vi "Read Port In.vi"(8 "error in (no error)":errorcluster caption="错误输入（无错误）", 10 "in_port":u16, 11 "dev":i32) -> (0 "error out":errorcluster caption="错误输出", 2 "in_port out":u16, 3 "function return":i32)   [LabVIEW 2018, in "恒凯采集卡.lvlib"]
doc: "int Read_Port_In(int dev,unsigned short* in_port);"
uses:
  data/Usb_Daq_V52_32.dll
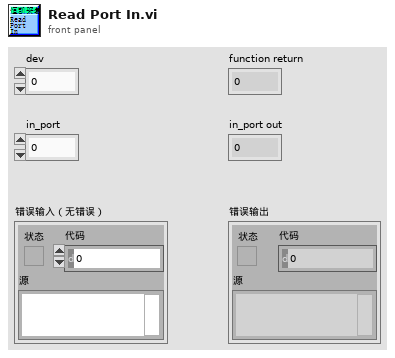
[diagram p1: front panel]
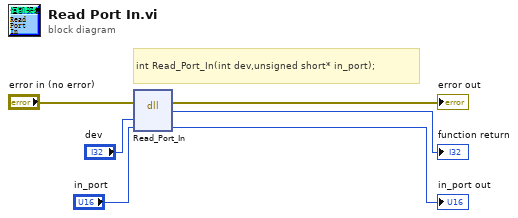
[diagram p0: block diagram]
diagram:
  # "int Read_Port_In(int dev,unsigned short* in_port);"
  n1 = dll-call lib="D:/ProgramFiles/NI/LabVIEW 2018/user.lib/Usb_Daq_V52_32/Usb_Daq_V52_32.*" fn="Read_Port_In"(error in="error in (no error)", "dev"="dev", "in_port"="in_port") -> (error out=→"error out":errorcluster, →"function return":i32, "in_port"=→"in_port out":u16)  [unwired: 3 in, 1 out]
